vi "example_usb.vi"() -> ()   [LabVIEW 2012, in "libirimager_direct_binding.lvlib"]
uses:
  libirimager_direct_binding.lvlib
panel:
  in  "Focus Pos %":sgl min=0 max=100
  in  "setFocusPos":bool
  out "function return setFocusPos":i32
  out "function return set radiation":i32
  in  "tAmbient":sgl=-999.9 format="%#_6f"
  in  "transmissivity(0..1)":sgl=1.0 format="%#_6f"
  in  "emissivity(0..1)":sgl=1.0 format="%#_6f"
  in  "setRadiation":bool
  in  "STOP":bool
  out "Thermal Image":picture
  out "function return thm":i32
  out "thermal data out":u16[](array[numeric])
  out "function return savepng":i32
  in  "triggerFlag":bool
  out "function return triggerAutoflag":i32
  in  "set_trigger_mode":bool
  in  "state":i32
  out "function return setAutoflag":i32
  in  "terminate":bool
  out "function return terminate":i32
  in  "getThm":bool
  in  "connect_usb":bool
  in  "xml_camera_config":string="generic.xml"
  out "function return":i32
  out "w out":i32
  out "h out":i32
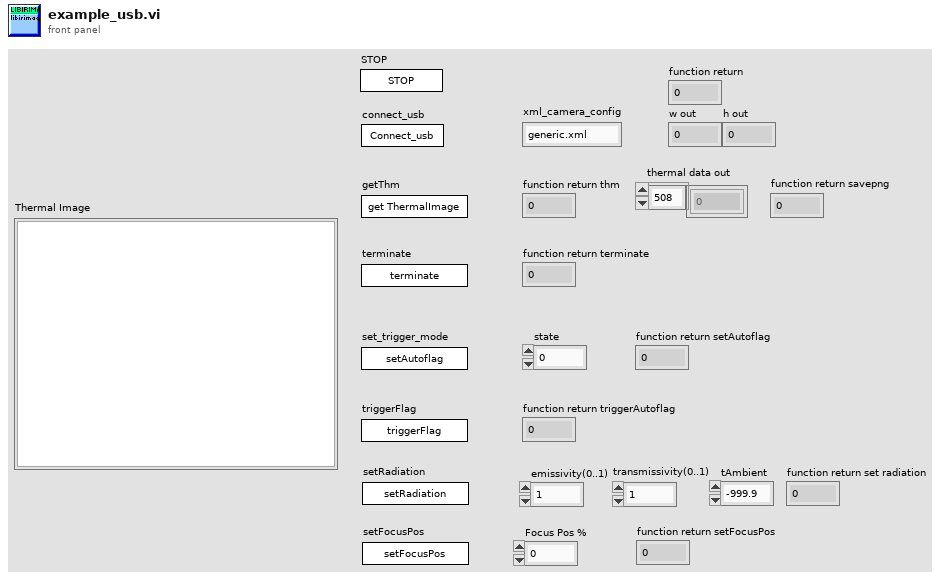
[diagram p1: front panel]
types:
  T1 = typedef "imagedata.ctl" = cluster{"image type":i32, "image depth":i32, "image":u8[], "mask":u8[], "colors":u32[], "Rectangle":cluster{"left":i16, "top":i16, "right":i16, "bottom":i16}}
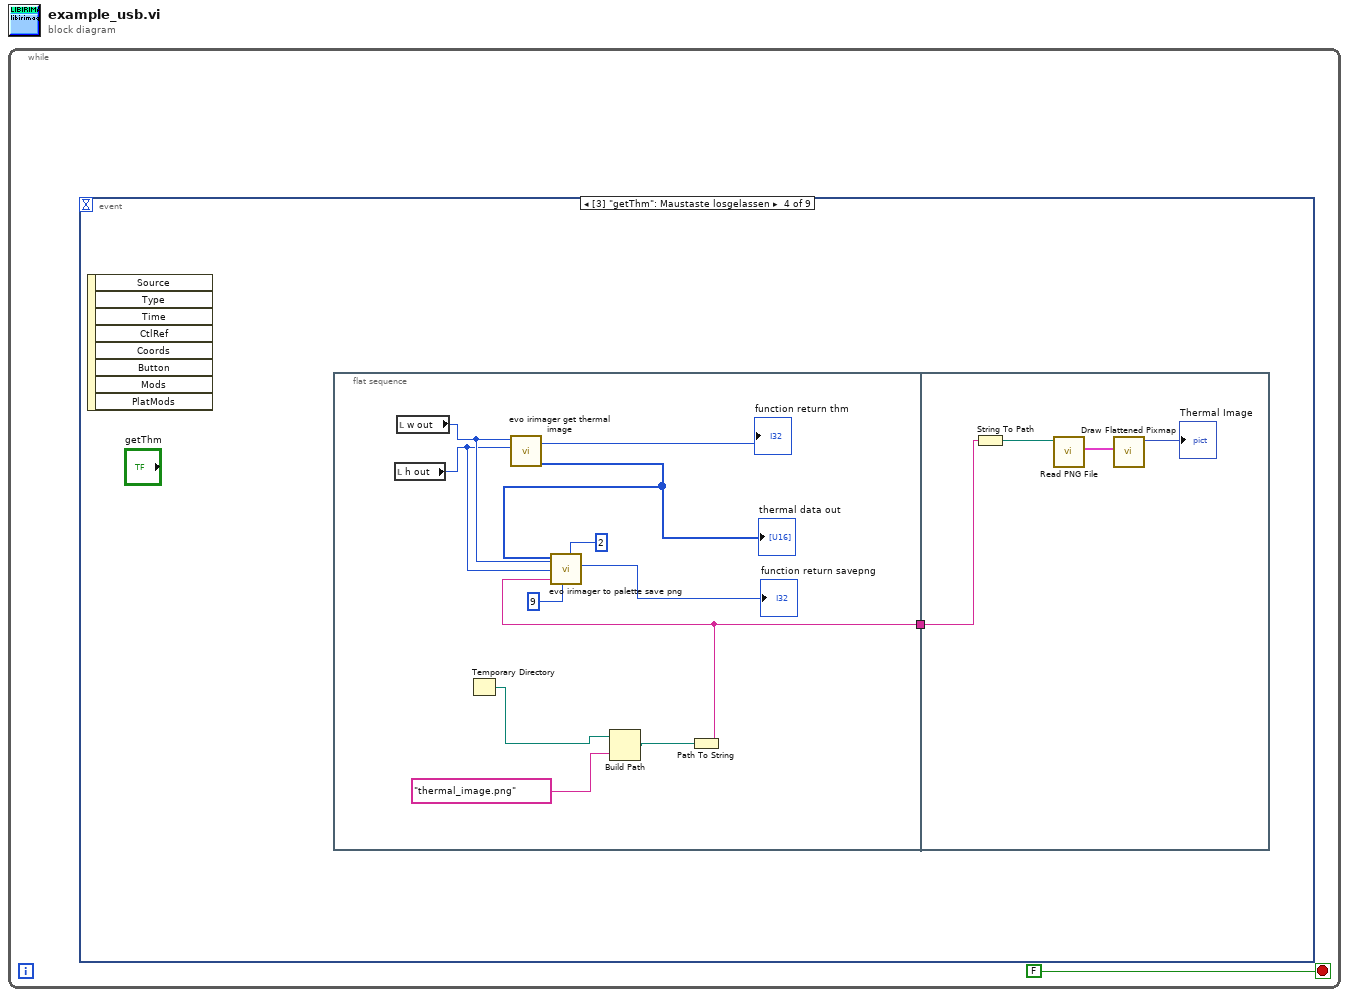
[diagram p0: block diagram]
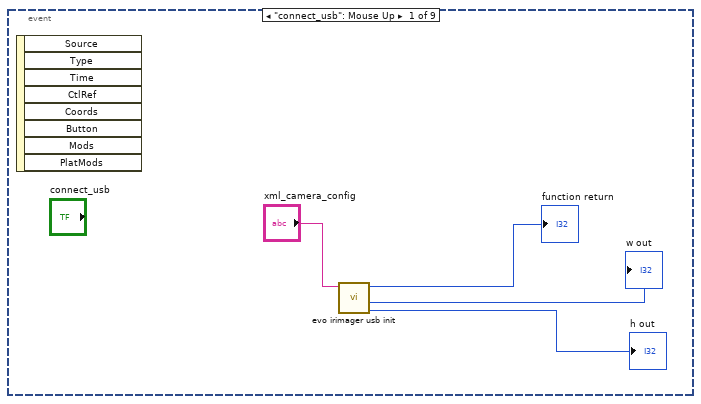
[diagram p2: hidden frame]
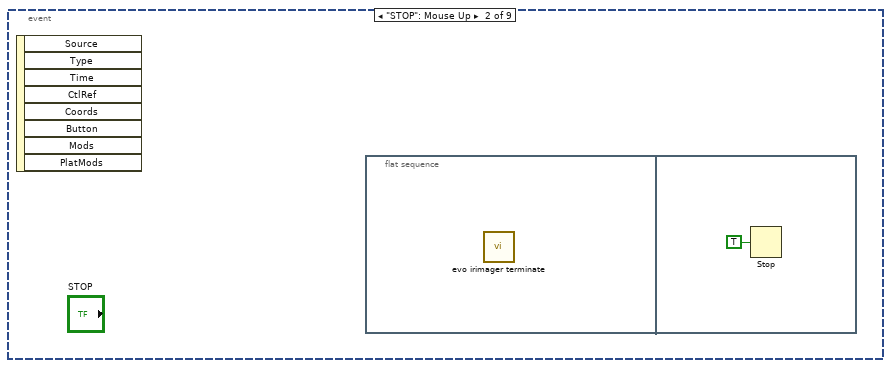
[diagram p3: hidden frame]
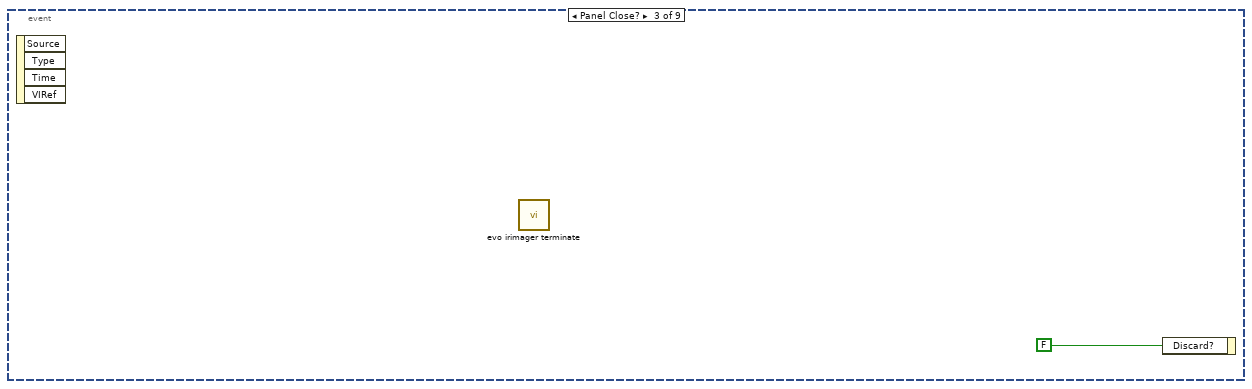
[diagram p4: hidden frame]
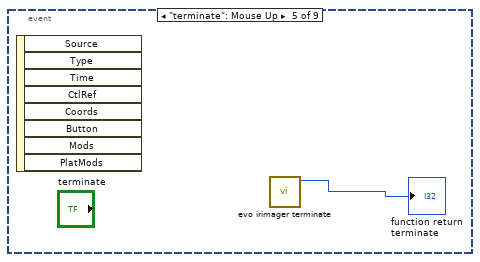
[diagram p5: hidden frame]
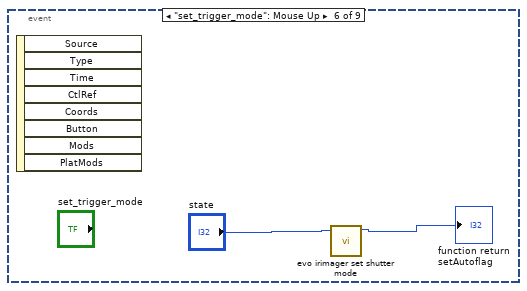
[diagram p6: hidden frame]
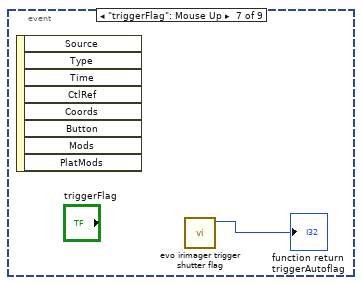
[diagram p7: hidden frame]
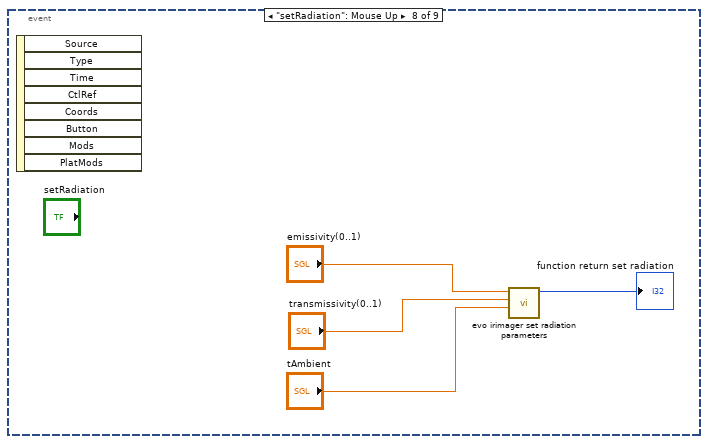
[diagram p8: hidden frame]
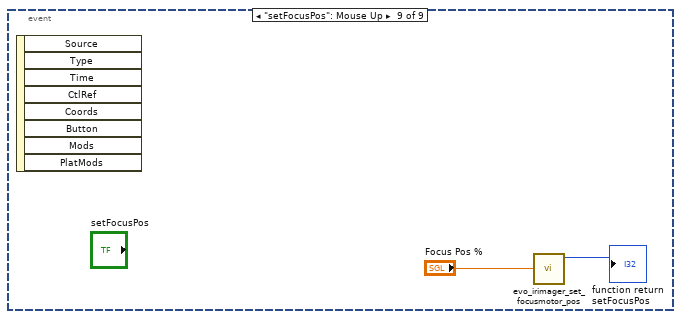
[diagram p9: hidden frame]
diagram:
  n1 = while {
    stop <- FALSE stop-if-true
    n2 = event shown="[3] \"getThm\": Maustaste losgelassen" {
      selector: _ -> [_ _ _ _ _ _ _ _ _]
      dyn-events: _ -> [_ _ _ _ _ _ _ _ _]
      timeout: _ -> [_ _ _ _ _ _ _ _ _]
      event "connect_usb": Mouse Up {
        n3 = event-data() -> ()  [unwired: 1 in, 8 out]
        n4 = call "evo irimager usb init.vi"("xml_config"="xml_camera_config") -> ("h out"=→"h out":i32, "w out"=→"w out":i32, "function return 2"=→"function return":i32)  [unwired: 7 in, 1 out]
      }
      event "STOP": Mouse Up {
        n5 = event-data() -> ()  [unwired: 1 in, 8 out]
        n6 = flat-sequence {
          frame #0 {
            n7 = call "evo irimager terminate.vi"() -> ()  [unwired: 11 in, 1 out]
          }
          frame #1 {
            n8 = Stop(stop? (T)=TRUE ("Stopp? (T)")) -> ()
          }
        }
      }
      event Panel Close? {
        n9 = event-data() -> ()  [unwired: 1 in, 4 out]
        n10 = call "evo irimager terminate.vi"() -> ()  [unwired: 11 in, 1 out]
        n11 = event-data("Discard?"=FALSE ("Verwerfen?")) -> ()  [unwired: 1 in, 1 out]
      }
      event "getThm": Mouse Up {
        n12 = event-data() -> ()  [unwired: 1 in, 8 out]
        n13 = flat-sequence {
          tunnel: [w11] -> w8
          tunnel: w8 -> [w20]
          frame #0 {
            n14 = local read "h out"() -> (w16:i32)
            n15 = local read "w out"() -> (w17:i32)
            n16 = Temporary Directory() -> (w10:path)
            n17 = call "evo irimager get thermal image.vi"("h"=w16, "w"=w17) -> ("data out"=w18:u16[], "function return"=→"function return thm":i32)  [unwired: 6 in, 2 out]
            "thermal data out" <- w18
            n18 = Build Path(base path=w10, name or relative path="thermal_image.png" ("String")) -> (appended path=w9:path)
            n19 = Path To String(path=w9) -> (string=w11:string)
            n20 = call "evo irimager to palette save png.vi"("palette_scale"=2, "palette"=9, "path"=w11, "h"=w16, "w"=w17, "thermal_data"=w18) -> ("function return"=→"function return savepng":i32)  [unwired: 4 in, 1 out]
          }
          frame #1 {
            n21 = String To Path(string=w20) -> (path=w21:path)
            n22 = call <vilib>:"Read PNG File.vi"("path to PNG file"=w21) -> ("image data"=w22:T1)  [unwired: 8 in, 2 out]
            n23 = call <vilib>:"Draw Flattened Pixmap.vi"("image data"=w22) -> ("new picture"=→"Thermal Image":picture)  [unwired: 8 in]
          }
        }
      }
      event "terminate": Mouse Up {
        n24 = event-data() -> ()  [unwired: 1 in, 8 out]
        n25 = call "evo irimager terminate.vi"() -> ("function return"=→"function return terminate":i32)  [unwired: 11 in]
      }
      event "set_trigger_mode": Mouse Up {
        n26 = event-data() -> ()  [unwired: 1 in, 8 out]
        n27 = call "evo irimager set shutter mode.vi"("mode"="state") -> ("function return"=→"function return setAutoflag":i32)  [unwired: 10 in]
      }
      event "triggerFlag": Mouse Up {
        n28 = event-data() -> ()  [unwired: 1 in, 8 out]
        n29 = call "evo irimager trigger shutter flag.vi"() -> ("function return"=→"function return triggerAutoflag":i32)  [unwired: 11 in]
      }
      event "setRadiation": Mouse Up {
        n30 = event-data() -> ()  [unwired: 1 in, 8 out]
        n31 = call "evo irimager set radiation parameters.vi"("tAmbient"="tAmbient", "transmissivity"="transmissivity(0..1)", "emissivity"="emissivity(0..1)") -> ("function return"=→"function return set radiation":i32)  [unwired: 8 in]
      }
      event "setFocusPos": Mouse Up {
        n32 = event-data() -> ()  [unwired: 1 in, 8 out]
        n33 = call "evo_irimager_set_focusmotor_pos.vi"("Focus Pos %"="Focus Pos %") -> ("function return"=→"function return setFocusPos":i32)  [unwired: 10 in]
      }
    }
  }
